vi "Client Println Test.vi"() -> ()   [LabVIEW 2014, in "ESP8266 WiFi Wrapper.lvlib"]
uses:
  ESP8266 WiFi Wrapper.lvlib
panel:
  in  "Input String":string="Hello world!"
  out "Error Out":errorcluster
  in  "Error In":errorcluster
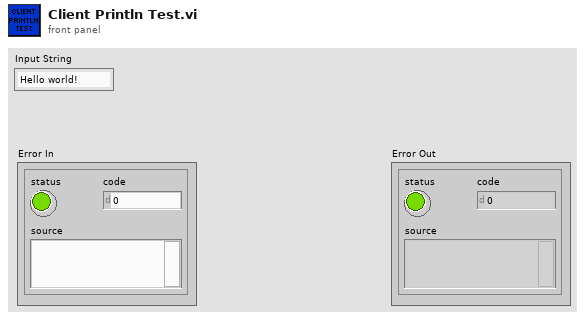
[diagram p1: front panel]
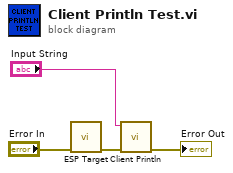
[diagram p0: block diagram]
diagram:
  n1 = call "ESP Target.vi"("Error In"="Error In") -> ("Error Out"=w2:errorcluster)  [unwired: 10 in]
  n2 = call "Client Println.vi"("Error In"=w2, "Input String"="Input String") -> ("Error Out"=→"Error Out":errorcluster)  [unwired: 9 in]
